vi "Formato data sql.vi"(11 "gg/mm/aaa":string) -> (3 "String":string)   [LabVIEW 2019]
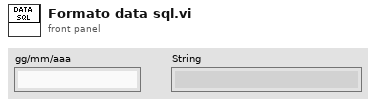
[diagram p1: front panel]
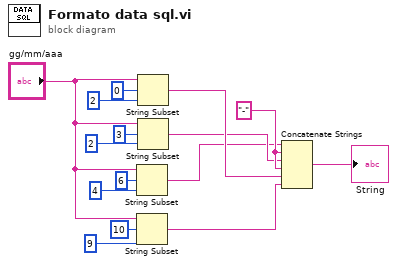
[diagram p0: block diagram]
diagram:
  w12 = "-" ("string")
  n1 = String Subset(string="gg/mm/aaa", offset (0)=6, length (rest)=4 ("length (rest)")) -> (substring=w10:string)
  n2 = String Subset(string="gg/mm/aaa", offset (0)=10, length (rest)=9 ("length (rest)")) -> (substring=w14:string)
  n3 = String Subset(string="gg/mm/aaa", offset (0)=0, length (rest)=2 ("length (rest)")) -> (substring=w13:string)
  n4 = String Subset(string="gg/mm/aaa", offset (0)=3, length (rest)=2 ("length (rest)")) -> (substring=w11:string)
  n5 = Concatenate Strings(w10, w12, w11, w12, w13, w14) -> (→"String":string)
